vi "Ionizer_Monitor.vi"() -> ()   [LabVIEW 2016]
panel:
  in  "Tab Control":T1(tab)
  out "Oven PS Current Actual":dbl
  out "Oven PS Voltage Actual":dbl
  out "Oven PS Current Set":dbl
  out "Oven PS Voltage Set":dbl
  out "Ionizer PS Current Actual":dbl
  out "Ionizer PS Voltage Actual":dbl
  out "Ionizer PS Current Set":dbl
  out "Ionizer PS Voltage Set":dbl
  out "Oven Temp":dbl
  in  "stop":bool
  out "Ionizer PS Current Actual":dbl(graph)
  out "Oven PS Current Actual":i32(graph)
  out "Oven Temperature":dbl(graph)
  out "Oven PS Voltage Actual":i32(graph)
  out "Ionizer PS Voltage Actual":dbl(graph)
  in  "Ionizer VISA resource":refnum<visa-resource-name>="TCPIP0::192.168.1.160::966::SOCKET"
  in  "Loop multiple (ms)":u32=500
  in  "Wait (ms)":u32=500
  in  "byte count":u32=15
  in  "Omega VISA resource":refnum<visa-resource-name>="TCPIP0::192.168.1.160::966::SOCKET"
  in  "Oven PS VISA resource":refnum<visa-resource-name>="TCPIP0::192.168.1.160::966::SOCKET"
  in  "byte count 3":u32=40
  in  "Loop multiple (ms) 2":u32=500
  out "Omega T error":errorcluster
  out "Ionizer Error":errorcluster
  out "Read errors":i32
  out "Oven PS Error":errorcluster
  out "Ionizer Iteration":i32
  out "Omega Iteration":i32
  out "Oven PS Iteration":i32
  out "Omega read buffer":string
  out "Oven PS read buffer":string
  # "°F"
  # "A"
  # "A"
  # "V"
  # "V"
  # "A"
  # "A"
  # "V"
  # "V"
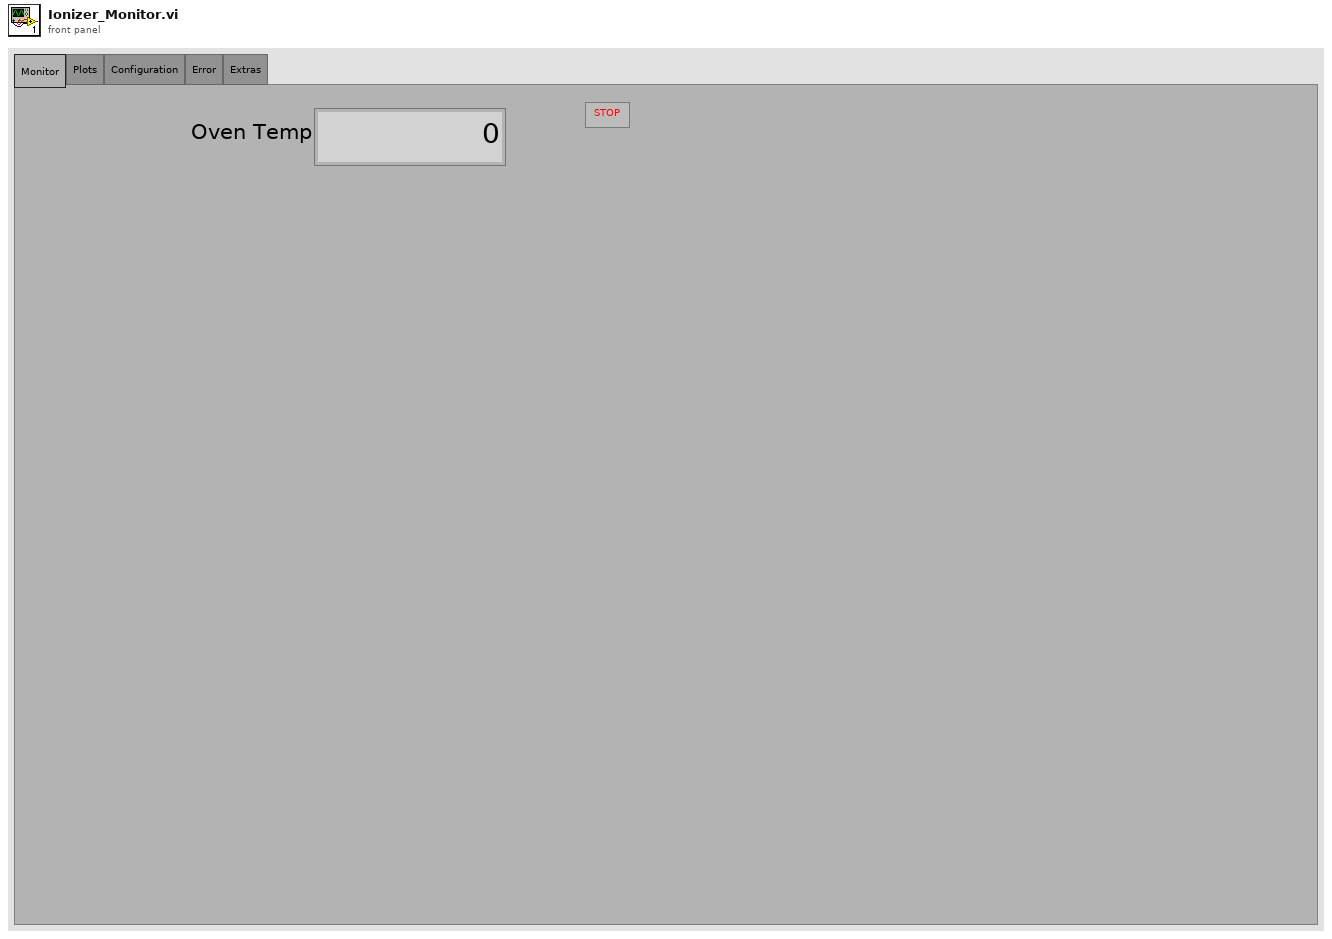
[diagram p1: front panel]
types:
  T1 = enum32{"Monitor", "Plots", "Configuration", "Error", "Extras"}
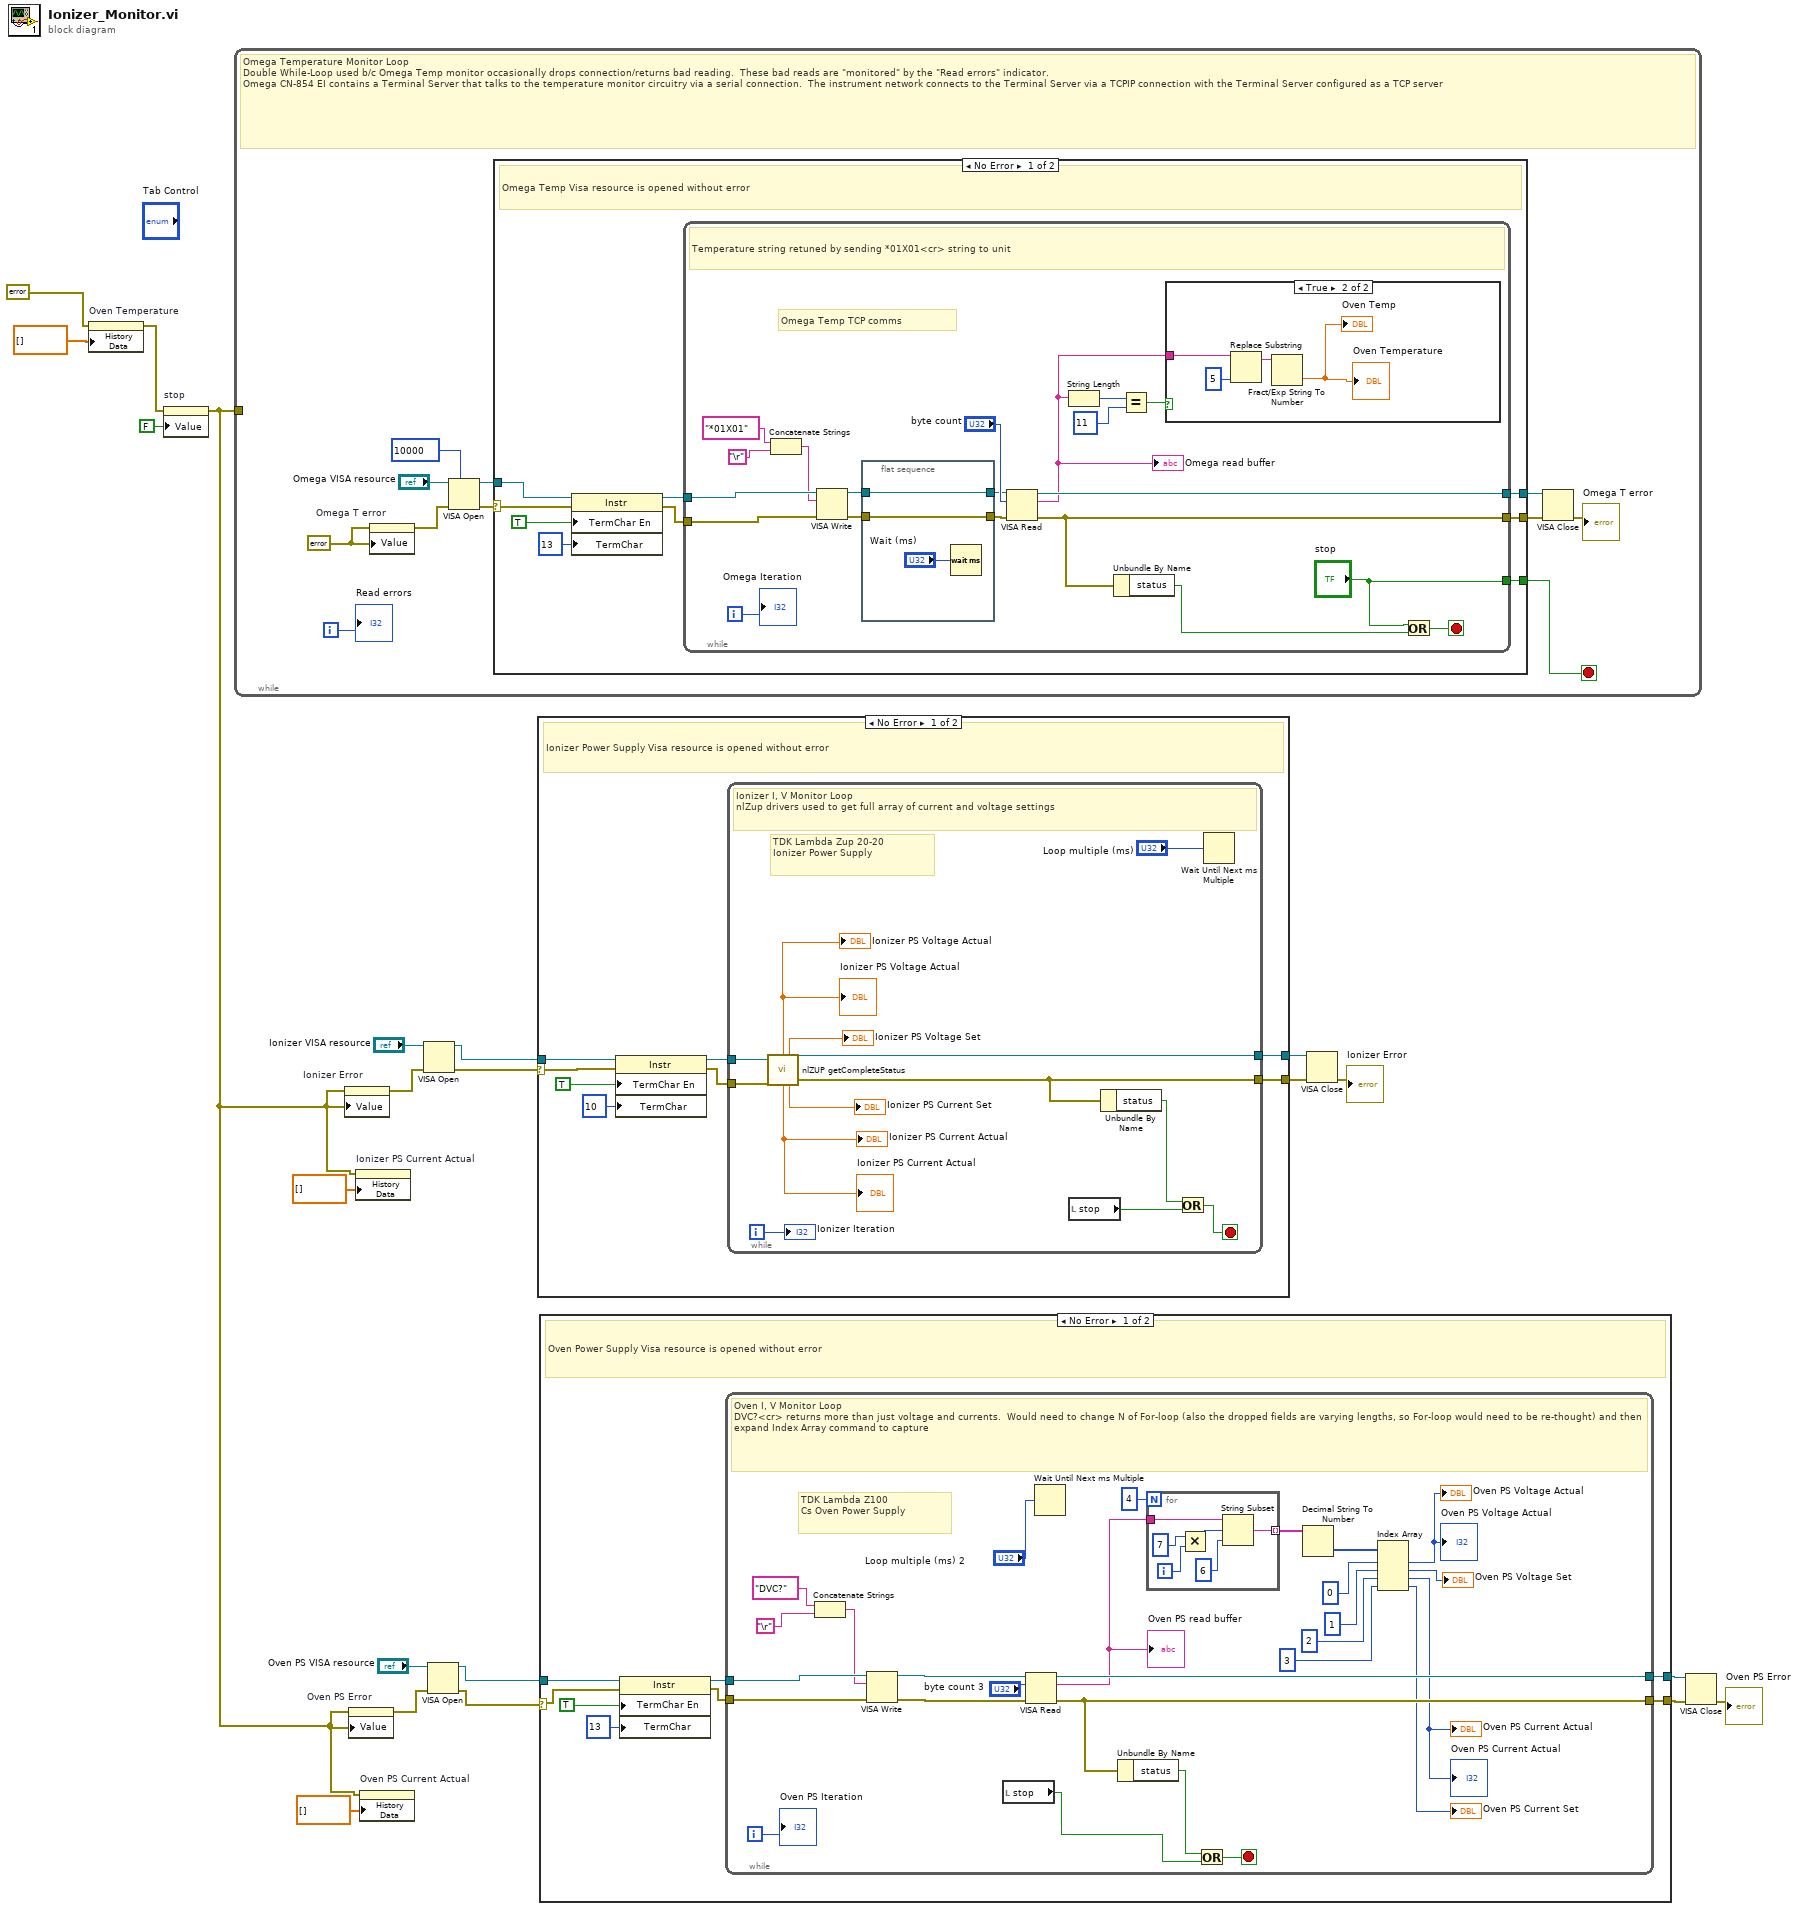
[diagram p0: block diagram]
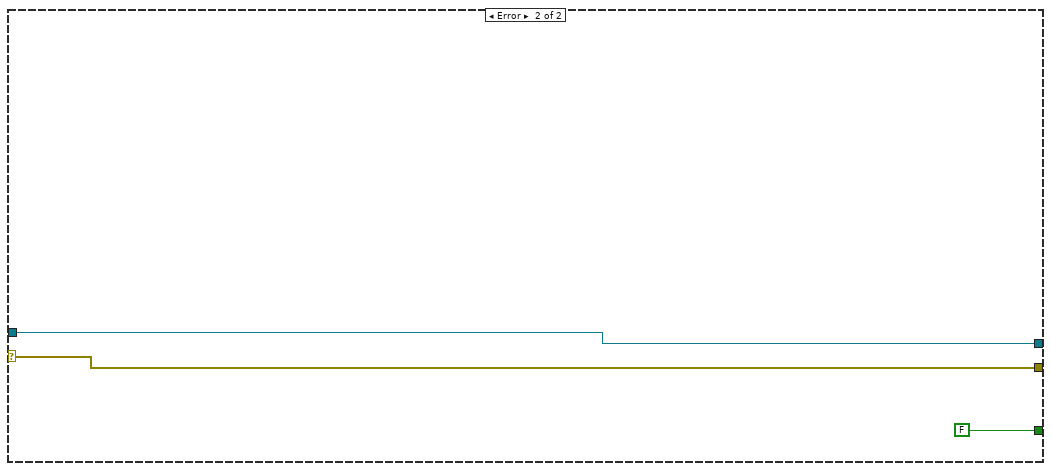
[diagram p5: hidden frame]
diagram:
  n1 = property on="Oven Temperature" class="WFChart (strict)"(error in=errorcluster {"status"=FALSE, "code"=0, "source"=""} ("error in (no error)"), "History Data"=dbl[] []) -> (error out=w12:errorcluster)  [unwired: 1 in, 1 out]
  n2 = property on="stop" class="Bool (strict)"(error in=w12, "Value"=FALSE ("stop")) -> (error out=w3:errorcluster)  [unwired: 1 in, 1 out]
  n3 = while {
    tunnel: w3 -> [_]
    i -> [w23]
    stop <- w24 stop-if-true
    w26 = errorcluster {"status"=FALSE, "code"=0, "source"=""} ("error in (no error)")
    # "Omega Temperature Monitor Loop\nDouble While-Loop used b/c Omega Temp monitor occasionally drops connection/returns bad reading.  These bad reads are \"monitored\" by the \"Read errors\" indicator.\nOmega CN-854 EI contains a Terminal Server that talks to the temperature monitor circuitry via a serial connection.  The instrument network connects to the Terminal Server via a TCPIP connection with the Terminal Server configured as a TCP server"
    n4 = property on="Omega T error" class="Clust (strict)"(error in=w26, "Value"=w26) -> (error out=w28:errorcluster)  [unwired: 1 in, 1 out]
    n5 = VISA Open(timeout (0)=u32 10000 ("VISA Open timeout (0)"), error in (no error)=w28, VISA resource name="Omega VISA resource") -> (VISA resource name=w32:refnum<visa-resource-name>, error out=w22:errorcluster)  [unwired: 2 in]
    n6 = case shown="No Error" w22 {
      selector: w22 -> [w34 w69]
      tunnel: w32 -> [w39 w71]
      tunnel: [w41 w71] -> w31
      tunnel: [w40 w69] -> w30
      tunnel: [w35 FALSE ("stop")] -> w24
      frame No Error {
        # "Omega Temp Visa resource is opened without error"
        n7 = property class="Instr"(reference=w39, error in=w34, "TermChar En"=TRUE ("Message Based Settings:Termination Character Enable"), "TermChar"=u8 13 ("Message Based Settings:Termination Character")) -> (reference out=w38:refnum<visa-resource-name>, error out=w33:errorcluster)
        n8 = while {
          tunnel: w38 -> [w57]
          tunnel: [w61] -> w41
          tunnel: w33 -> [w52]
          tunnel: [w60] -> w40
          tunnel: ["stop"] -> w35
          i -> [w58]
          stop <- w59 stop-if-true
          # "Omega Temp TCP comms"
          # "Temperature string retuned by sending *01X01<cr> string to unit"
          n9 = Concatenate Strings("*01X01" ("data in"), "\r") -> (w54:string)
          n10 = VISA Write(VISA resource name=w57, write buffer=w54, error in (no error)=w52) -> (VISA resource name out=w45:refnum<visa-resource-name>, error out=w47:errorcluster)  [unwired: 1 out]
          n11 = flat-sequence {
            tunnel: w47 -> [w64]
            tunnel: [w64] -> w46
            tunnel: w45 -> [w63]
            tunnel: [w63] -> w44
            frame #0 {
              n12 = Wait (ms)(milliseconds to wait="Wait (ms)") -> ()  [unwired: 1 out]
            }
          }
          n13 = VISA Read(VISA resource name=w44, byte count="byte count", error in (no error)=w46) -> (VISA resource name out=w61:refnum<visa-resource-name>, read buffer=w48:string, error out=w60:errorcluster)  [unwired: 1 out]
          "Omega read buffer" <- w48
          n14 = String Length(string=w48) -> (length=w51:i32)
          n15 = Unbundle By Name(w60) -> ("status"=w43:bool)
          n16 = Equal?(x=w51, y=11) -> (x = y?=w49:bool)
          n17 = case shown="True" w49 {
            tunnel: w48 -> [_ w65]
            frame False {
            }
            frame True {
              n18 = Replace Substring(2:5 ("length (len. of substring)"), 5:w65) -> (1:w66:string)  [unwired: 2 in, 1 out]
              n19 = Fract/Exp String To Number(string=w66) -> (number=→"Oven Temp" →"Oven Temperature":dbl)  [unwired: 3 in, 1 out]
            }
          }
          n20 = Or(x="stop", y=w43) -> (x .or. y?=w59:bool)
          "Omega Iteration" <- w58
        }
      }
      frame Error {
      }
    }
    n21 = VISA Close(VISA resource name=w31, error in (no error)=w30) -> (error out=→"Omega T error":errorcluster)
    "Read errors" <- w23
  }
  n22 = property on="Ionizer Error" class="Clust (strict)"(error in=w3, "Value"=w3) -> (error out=w16:errorcluster)  [unwired: 1 in, 1 out]
  n23 = property on="Oven PS Error" class="Clust (strict)"(error in=w3, "Value"=w3) -> (error out=w6:errorcluster)  [unwired: 1 in, 1 out]
  n24 = property on="Ionizer PS Current Actual" class="WFChart (strict)"(error in=w3, "History Data"=dbl[] []) -> ()  [unwired: 1 in, 2 out]
  n25 = property on="Oven PS Current Actual" class="WFChart (strict)"(error in=w3, "History Data"=dbl[] []) -> ()  [unwired: 1 in, 2 out]
  n26 = VISA Open(error in (no error)=w16, VISA resource name="Ionizer VISA resource") -> (VISA resource name=w20:refnum<visa-resource-name>, error out=w1:errorcluster)  [unwired: 3 in]
  n27 = VISA Open(error in (no error)=w6, VISA resource name="Oven PS VISA resource") -> (VISA resource name=w10:refnum<visa-resource-name>, error out=w2:errorcluster)  [unwired: 3 in]
  n28 = case shown="No Error" w1 {
    selector: w1 -> [w72 w93]
    tunnel: w20 -> [w77 w94]
    tunnel: [w79 w94] -> w19
    tunnel: [w78 w93] -> w18
    frame No Error {
      # "Ionizer Power Supply Visa resource is opened without error"
      n29 = property class="Instr"(reference=w77, error in=w72, "TermChar En"=TRUE ("Message Based Settings:Termination Character Enable"), "TermChar"=u8 10 ("Message Based Settings:Termination Character")) -> (reference out=w76:refnum<visa-resource-name>, error out=w75:errorcluster)
      n30 = while {
        tunnel: w76 -> [w87]
        tunnel: [w85] -> w79
        tunnel: w75 -> [w86]
        tunnel: [w84] -> w78
        i -> [w89]
        stop <- w90 stop-if-true
        # "TDK Lambda Zup 20-20\nIonizer Power Supply"
        # "Ionizer I, V Monitor Loop\nnlZup drivers used to get full array of current and voltage settings"
        n31 = call <instrlib>:"nlZUP getCompleteStatus.vi"("VISA resource name"=w87, "error in (no error)"=w86) -> ("Actual Voltage"=→"Ionizer PS Voltage Actual" →"Ionizer PS Voltage Actual":dbl, "Voltage Setting"=→"Ionizer PS Voltage Set":dbl, "VISA resource name out"=w85:refnum<visa-resource-name>, "Actual Current"=→"Ionizer PS Current Actual" →"Ionizer PS Current Actual":dbl, "Current Setting"=→"Ionizer PS Current Set":dbl, "error out"=w84:errorcluster)  [unwired: 5 in, 3 out]
        n32 = local read "stop"() -> (w88:bool)
        n33 = Unbundle By Name(w84) -> ("status"=w91:bool)
        n34 = Or(x=w91, y=w88) -> (x .or. y?=w90:bool)
        n35 = Wait Until Next ms Multiple(millisecond multiple="Loop multiple (ms)") -> ()  [unwired: 1 out]
        "Ionizer Iteration" <- w89
      }
    }
    frame Error {
    }
  }
  n36 = case shown="No Error" w2 {
    selector: w2 -> [w95 w136]
    tunnel: w10 -> [w100 w137]
    tunnel: [w102 w137] -> w9
    tunnel: [w101 w136] -> w8
    frame No Error {
      # "Oven Power Supply Visa resource is opened without error"
      n37 = property class="Instr"(reference=w100, error in=w95, "TermChar En"=TRUE ("Message Based Settings:Termination Character Enable"), "TermChar"=u8 13 ("Message Based Settings:Termination Character")) -> (reference out=w99:refnum<visa-resource-name>, error out=w98:errorcluster)
      n38 = while {
        tunnel: w99 -> [w120]
        tunnel: [w127] -> w102
        tunnel: w98 -> [w126]
        tunnel: [w124] -> w101
        i -> [w121]
        stop <- w122 stop-if-true
        # "TDK Lambda Z100\nCs Oven Power Supply"
        # "Oven I, V Monitor Loop\nDVC?<cr> returns more than just voltage and currents.  Would need to change N of For-loop (also the dropped fields are varying lengths, so For-loop would need to be re-thought) and then expand Index Array command to capture"
        n39 = Concatenate Strings("DVC?" ("string"), "\r") -> (w116:string)
        n40 = VISA Write(VISA resource name=w120, write buffer=w116, error in (no error)=w126) -> (VISA resource name out=w128:refnum<visa-resource-name>, error out=w125:errorcluster)  [unwired: 1 out]
        n41 = local read "stop"() -> (w118:bool)
        n42 = VISA Read(VISA resource name=w128, byte count="byte count 3", error in (no error)=w125) -> (VISA resource name out=w127:refnum<visa-resource-name>, read buffer=w114:string, error out=w124:errorcluster)  [unwired: 1 out]
        "Oven PS read buffer" <- w114
        n43 = Wait Until Next ms Multiple(millisecond multiple="Loop multiple (ms) 2") -> ()  [unwired: 1 out]
        n44 = Unbundle By Name(w124) -> ("status"=w123:bool)
        n45 = for {
          N: 4 -> [_]
          tunnel: w114 -> [w135]
          tunnel: [w133] -> w104 mode=indexing
          i -> [w132]
          n46 = Multiply(x=7, y=w132) -> (x*y=w131:i32)
          n47 = String Subset(string=w135, offset (0)=w131, length (rest)=6 ("length (rest)")) -> (substring=w133:string)
        }
        n48 = Or(x=w123, y=w118) -> (x .or. y?=w122:bool)
        n49 = Decimal String To Number(string=w104) -> (number=w103:i32[])  [unwired: 2 in, 1 out]
        n50 = Index Array(array=w103, index #1=0 ("index"), index #2=1 ("index"), index #3=2 ("index"), index #4=3 ("index")) -> (element #1=→"Oven PS Voltage Actual" →"Oven PS Voltage Actual":i32, element #2=→"Oven PS Voltage Set":i32, element #3=→"Oven PS Current Actual" →"Oven PS Current Actual":i32, element #4=→"Oven PS Current Set":i32)
        "Oven PS Iteration" <- w121
      }
    }
    frame Error {
    }
  }
  n51 = VISA Close(VISA resource name=w19, error in (no error)=w18) -> (error out=→"Ionizer Error":errorcluster)
  n52 = VISA Close(VISA resource name=w9, error in (no error)=w8) -> (error out=→"Oven PS Error":errorcluster)
